vi "MotorMath.vi"(8 "x":dbl) -> (0 "output cluster":cluster{i32, "upper limit":dbl})   [LabVIEW 2012]
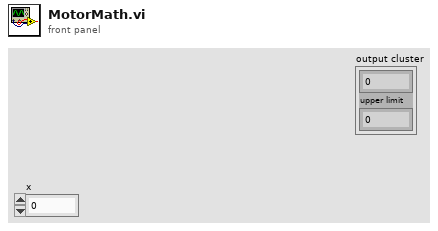
[diagram p1: front panel]
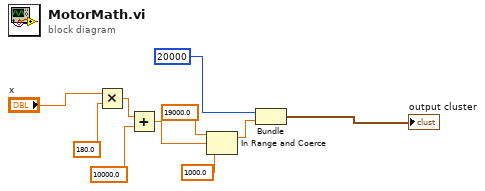
[diagram p0: block diagram]
diagram:
  n1 = Multiply(x="x", y=180.0) -> (x*y=w6:dbl)
  n2 = Add(x=w6, y=10000.0) -> (x+y=w3:dbl)
  n3 = In Range and Coerce(upper limit=19000.0, x=w3, lower limit=1000.0) -> (coerced(x)=w7:dbl)  [unwired: 1 out]
  n4 = Bundle(20000, "upper limit"=w7) -> (→"output cluster":cluster{i32, "upper limit":dbl})  [unwired: 1 in]
